vi "stop.vi"(8 "error in (no error)":errorcluster, 11 "DL090202FPGAClock in":refnum<class "ClockDL090202FPGA.lvclass">) -> (0 "error out":errorcluster, 3 "DL090202FPGAClock out":refnum<class "ClockDL090202FPGA.lvclass">)   [LabVIEW 2010, in "ClockDL090202FPGA.lvclass"]
uses:
  ClockDL090202FPGA.lvclass
  ClockDL090202FPGA.lvclass/ClockDL090202FPGA.ctl
  FPGAWrapper/GenericFPGAWrapper/GenericFPGAWrapper/GenericFPGAWrapper.lvclass
  common/classes/ErrorController/ErrorController/class_data.vi
  common/classes/ErrorController/ErrorController/ErrorController.lvclass
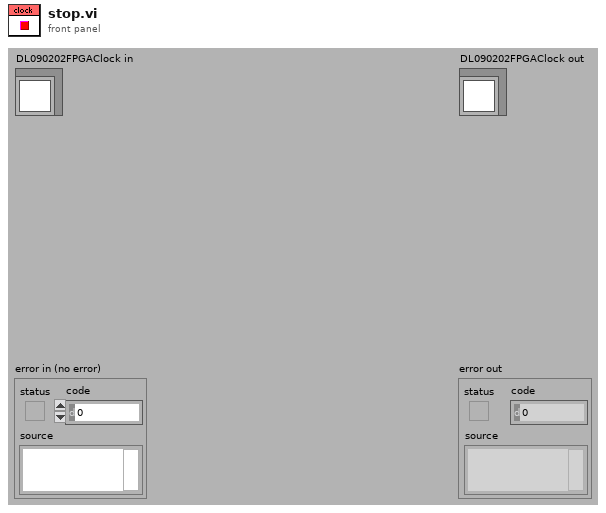
[diagram p1: front panel]
types:
  T1 = typedef "ClockDL090202FPGA.lvclass/type_enum.ctl" = enum16{"pixel clock", "gate 1", "gate 2", "gate 3"}
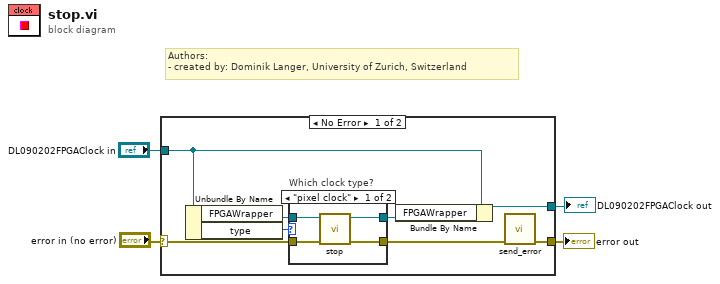
[diagram p0: block diagram]
diagram:
  # "Authors: \n- created by: Dominik Langer, University of Zurich, Switzerland"
  n1 = case shown="No Error" "error in (no error)" {
    selector: "error in (no error)" -> [w12 w20]
    tunnel: [w6 w20] -> w3
    tunnel: [w8 w19] -> w1
    tunnel: "DL090202FPGAClock in" -> [w9 w19]
    frame No Error {
      n2 = Unbundle By Name(w9) -> ("FPGAWrapper"=w11:refnum<class "GenericFPGAWrapper.lvclass">, "type"=w7:T1)
      n3 = case "Which clock type?" shown="\"pixel clock\"" w7 {
        tunnel: w12 -> [w16 w18]
        tunnel: [w15 w18] -> w5
        tunnel: w11 -> [w14 w17]
        tunnel: [w13 w17] -> w10
        frame "pixel clock" {
          n4 = call-dynamic "stop.vi"("error in (no error)"=w16, "GenericFPGAWrapper in"=w14) -> ("error out"=w15:errorcluster, "GenericFPGAWrapper out"=w13:refnum<class "GenericFPGAWrapper.lvclass">)  [unwired: 8 out]
        }
        frame Default {
        }
      }
      n5 = Bundle By Name(cluster=w9, "FPGAWrapper"=w10) -> (w8:refnum<class "ClockDL090202FPGA.lvclass">)
      n6 = call "send_error.vi"("error in (no error)"=w5) -> ("error out"=w6:errorcluster)  [unwired: 10 in]
    }
    frame Error {
    }
  }
  "error out" <- w3
  "DL090202FPGAClock out" <- w1
